vi "EscapeURI.vi"(11 "URI":string) -> (3 "Escaped URI":string)   [LabVIEW 2013, in "URI.lvlib"]
uses:
  URI.lvlib
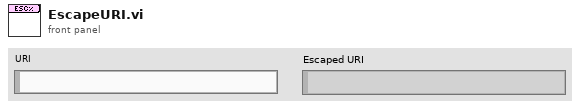
[diagram p1: front panel]
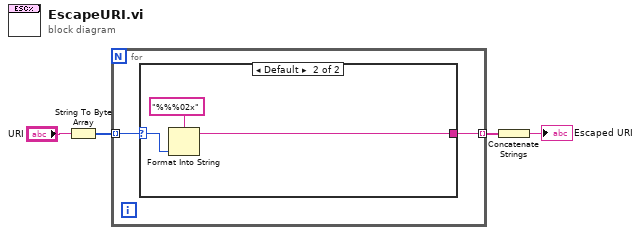
[diagram p0: block diagram]
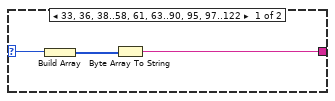
[diagram p2: hidden frame]
diagram:
  n1 = String To Byte Array(string="URI") -> (unsigned byte array=w3:u8[])
  n2 = for {
    tunnel: w3 -> [w6] mode=indexing
    tunnel: [w5] -> w2 mode=indexing
    n3 = case shown="Default" w6 {
      selector: w6 -> [w9 w12]
      tunnel: [w7 w10] -> w5
      frame 33, 36, 38..58, 61, 63..90, 95, 97..122 {
        n4 = Build Array(w9) -> (w8:u8[])
        n5 = Byte Array To String(unsigned byte array=w8) -> (string=w7:string)
      }
      frame Default {
        n6 = Format Into String(format string="%%%02x", w12) -> (resulting string=w10:string)  [unwired: 2 in, 1 out]
      }
    }
  }
  n7 = Concatenate Strings(w2) -> (→"Escaped URI":string)
